vi "Measure Intensity Dep.vi"(0 "User Name":string, 1 "Cell details cluster":T3={"Cell Position"=16, "Cell Label"="", "Pixel to measure"=0, "Area (cm^2)"=0.126, "Variable"="", "Variable value"="", "Scan settings in queue"=0, "Light or dark"="", "Measurement type"=""} {"Pixel to measure" items=["All", "1", "2", "3", "4", "5", "6", "7", "8"]}, 2 "Date array":string[](array[string]), 5 "Experiment Title":string, 9 "No. of Suns":dbl, 11 "error in (no error)":errorcluster, 12 "Scan settings":T1={"J-V scan"=TRUE, "J-t scan"=FALSE, "Min voltage (V)"=0.0, "Max voltage (V)"=1.4, "Step (V)"=0.01, "Measurement delay (ms)"=10.0, "1st scan FB-SC"=TRUE, "Inverted structure"=FALSE, "Stabilisation time (s)"=0.0, "Stabilisation mode"=0, "Stabilisation value (V or A) "=0.0, "Step time (s)"=1.0, "Integration time"=0, "Repeat light scans"=FALSE, "Stabilisation in the dark?"=FALSE, "J-t Min (V)"=0.0, "J-t Max (V)"=1.4, "J-t Step (V)"=0.01, "Max. power stabilisation"=FALSE, "J-t 1st scan FB-SC"=TRUE, "J-t Inverted structure"=FALSE, "Max power tracking"=FALSE, "Vmp (V)"=0.7, "Total stabilisation time (s)"=100.0, "J-t best pixel only"=0, "Max power best pixel only"=0, "Vmp from J-V scan"=FALSE, "Intensity dependence"=FALSE, "P dep best pixel only"=0, "External quantum efficiency"=FALSE, "EQE best pixel only"=0, "WL min (nm)"=300.0, "WL max (nm)"=900.0, "WL step (nm)"=5.0, "Wait (ms)"=100.0, "No. of repeat scans"=2.0, "Only repeat for best pixel"=0, "Chopper Freq.  (Hz)"=90.0, "Time Constant (s)"=2.0, "Stabilisation time step (s)"=1.0, "Illumination conditions"=2, "Scan rate min (V/s)"=0.1, "Scan rate max (V/s)"=1.0, "No. of scan rate steps"=1.0, "Scan rate voltage step priority"=FALSE, "Scan rate measurement delay priority"=FALSE, "J-t Illumination conditions"=0, "White bias  (no. of suns)"=200.0, "Max P stab. Specific voltage"=FALSE} {"J-t Illumination conditions" items=["Light only", "Dark only", "Light then dark", "Dark then light"]; "No. of scan rate steps" min=1.0 step=1.0; "Illumination conditions" items=["Light only", "Dark only", "Light then dark", "Dark then light", "Light then dark then light", "Dark then light then dark"]; "Time Constant (s)" items=["0.003", "0.01", "0.03", "0.1", "0.3", "1", "3", "10", "30", "100"]; "Only repeat for best pixel" items=["only for best pixel", "for best 2 pixels", "for best 3 pixels", "for best 4 pixels", "for best 5 pixels", "for best 6 pixels", "for best 7 pixels", "for all pixels"]; "No. of repeat scans" min=1.0 step=1.0; "EQE best pixel only" items=["only the best pixel", "the best 2 pixel", "the best 3 pixel", "the best 4 pixel", "the best 5 pixel", "the best 6 pixel", "the best 7 pixel", "all pixels"]; "P dep best pixel only" items=["only the best pixel", "the best 2 pixels", "the best 3 pixels", "the best 4 pixels", "the best 5 pixels", "the best 6 pixels", "the best 7 pixels", "all pixels"]; "Max power best pixel only" items=["only the best pixel", "the best 2 pixels", "the best 3 pixels", "the best 4 pixels", "the best 5 pixels", "the best 6 pixels", "the best 7 pixels", "all pixels"]; "J-t best pixel only" items=["only the best pixel", "the best 2 pixels", "the best 3 pixels", "the best 4 pixels", "the best 5 pixels", "the best 6 pixels", "the best 7 pixels", "all pixels"]; "Integration time" items=["Fast", "Normal", "High Accuracy"]; "Stabilisation mode" items=["V", "I"]; "Measurement delay (ms)" min=10.0}, 13 "Scan rate (V/s)":dbl, 14 "Skip pixel?":bool) -> (4 "JV Curve":cluster{"Y":dbl[], "Y":dbl[]}[](graph), 15 "Log Table":string[][](table))   [LabVIEW 2016]
uses:
  TypeDefs/NPLC for JV scan.ctl
  <instrlib>/keithley_24xx/Keithley 24XX/Public/Data/Read (Single Point).vi
  TypeDefs/Settings Boolean.ctl
  TypeDefs/Scan settings.ctl
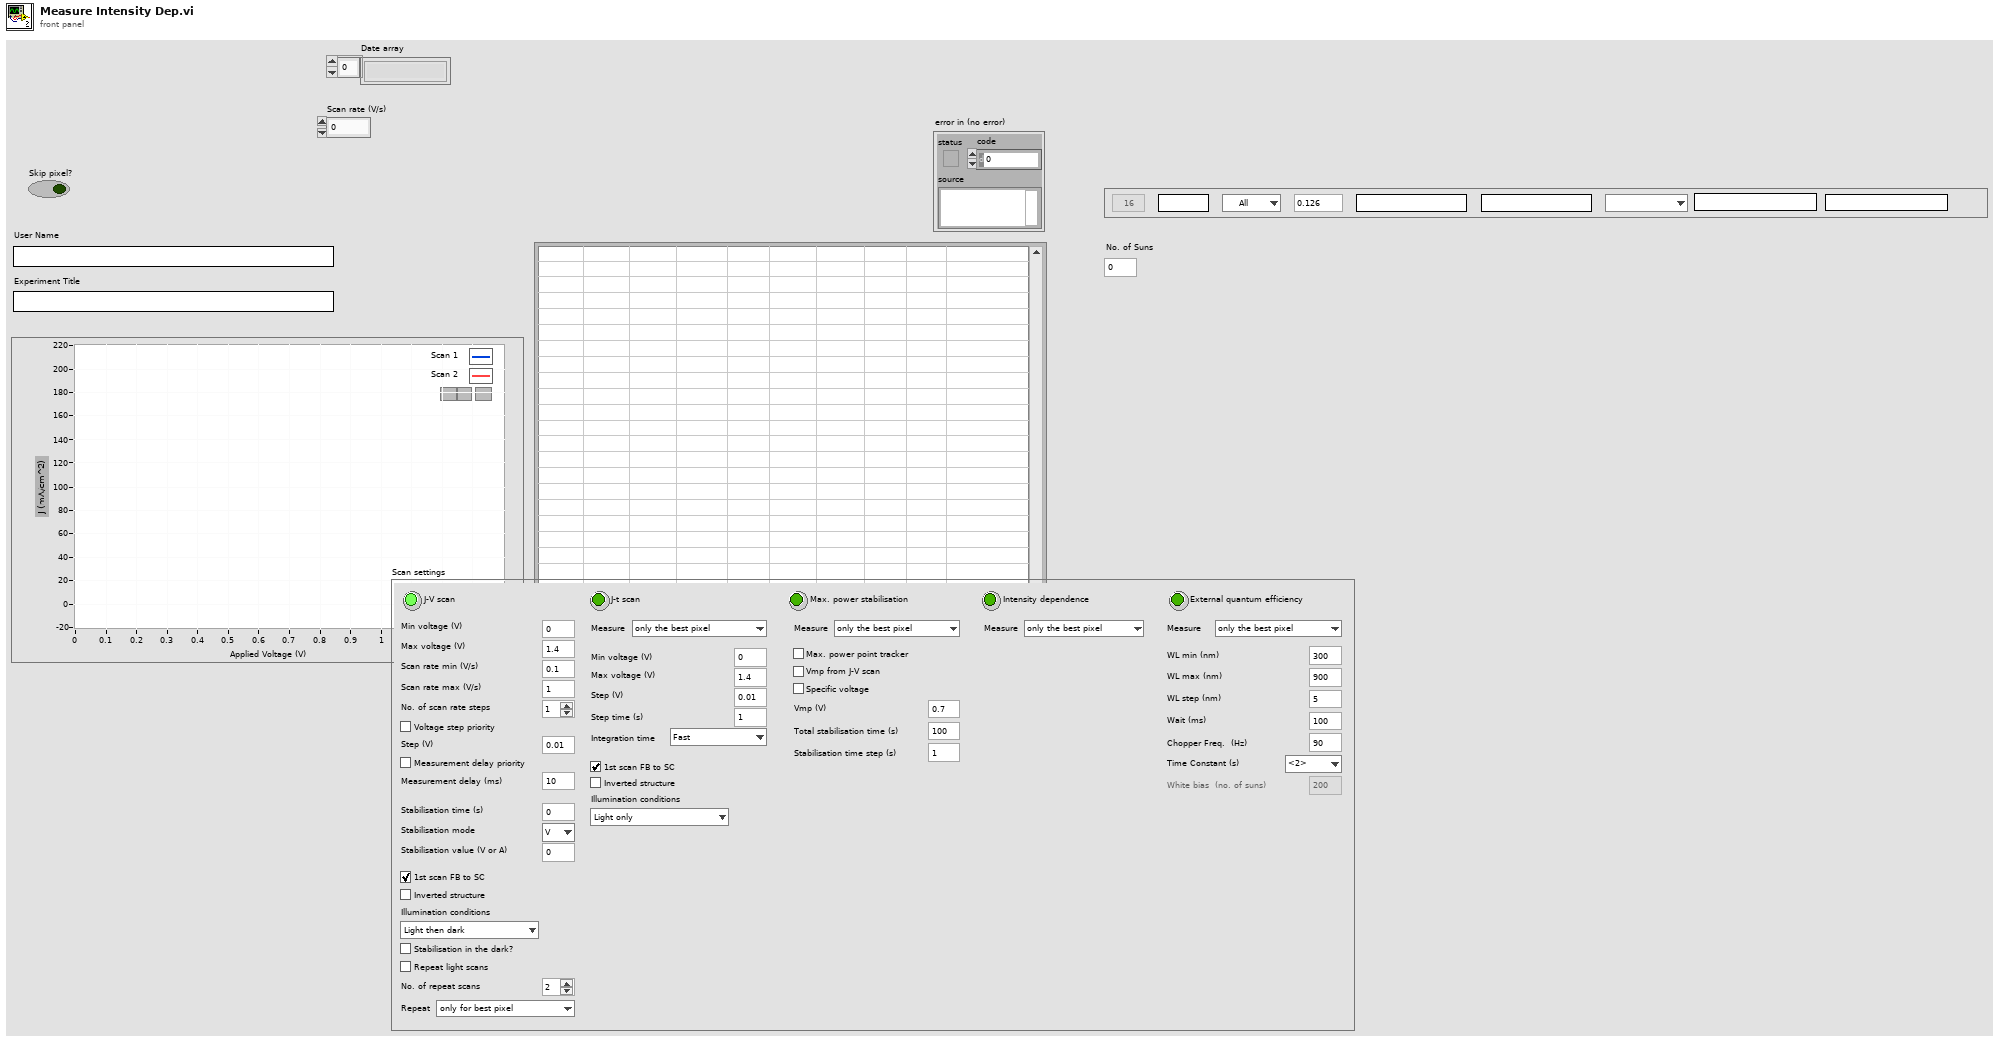
[diagram p1: front panel]
types:
  T1 = typedef "Scan settings.ctl" = cluster{"J-V scan":T2, "J-t scan":bool, "Min voltage (V)":dbl, "Max voltage (V)":dbl, "Step (V)":dbl, "Measurement delay (ms)":dbl, "1st scan FB-SC":bool, "Inverted structure":bool, "Stabilisation time (s)":dbl, "Stabilisation mode":u16, "Stabilisation value (V or A) ":dbl, "Step time (s)":dbl, "Integration time":u16, "Repeat light scans":bool, "Stabilisation in the dark?":bool, "J-t Min (V)":dbl, "J-t Max (V)":dbl, "J-t Step (V)":dbl, "Max. power stabilisation":bool, "J-t 1st scan FB-SC":bool, "J-t Inverted structure":bool, "Max power tracking":bool, "Vmp (V)":dbl, "Total stabilisation time (s)":dbl, "J-t best pixel only":u16, "Max power best pixel only":u16, "Vmp from J-V scan":bool, "Intensity dependence":bool, "P dep best pixel only":u16, "External quantum efficiency":bool, "EQE best pixel only":u16, "WL min (nm)":dbl, "WL max (nm)":dbl, "WL step (nm)":dbl, "Wait (ms)":dbl, "No. of repeat scans":dbl, "Only repeat for best pixel":u16, "Chopper Freq.  (Hz)":dbl, "Time Constant (s)":dbl, "Stabilisation time step (s)":dbl, "Illumination conditions":u16, "Scan rate min (V/s)":dbl, "Scan rate max (V/s)":dbl, "No. of scan rate steps":dbl, "Scan rate voltage step priority":bool, "Scan rate measurement delay priority":bool, "J-t Illumination conditions":u16, "White bias  (no. of suns)":dbl, "Max P stab. Specific voltage":bool}
  T2 = typedef "Settings Boolean.ctl" = bool
  T3 = cluster{"Cell Position":i32, "Cell Label":string, "Pixel to measure":u16, "Area (cm^2)":dbl, "Variable":string, "Variable value":string, "Scan settings in queue":u16, "Light or dark":string, "Measurement type":string}
  T4 = typedef "NPLC for JV scan.ctl" = dbl
  T5 = typedef "imagedata.ctl" = cluster{"image type":i32, "image depth":i32, "image":u8[], "mask":u8[], "colors":u32[], "Rectangle":cluster{"left":i16, "top":i16, "right":i16, "bottom":i16}}
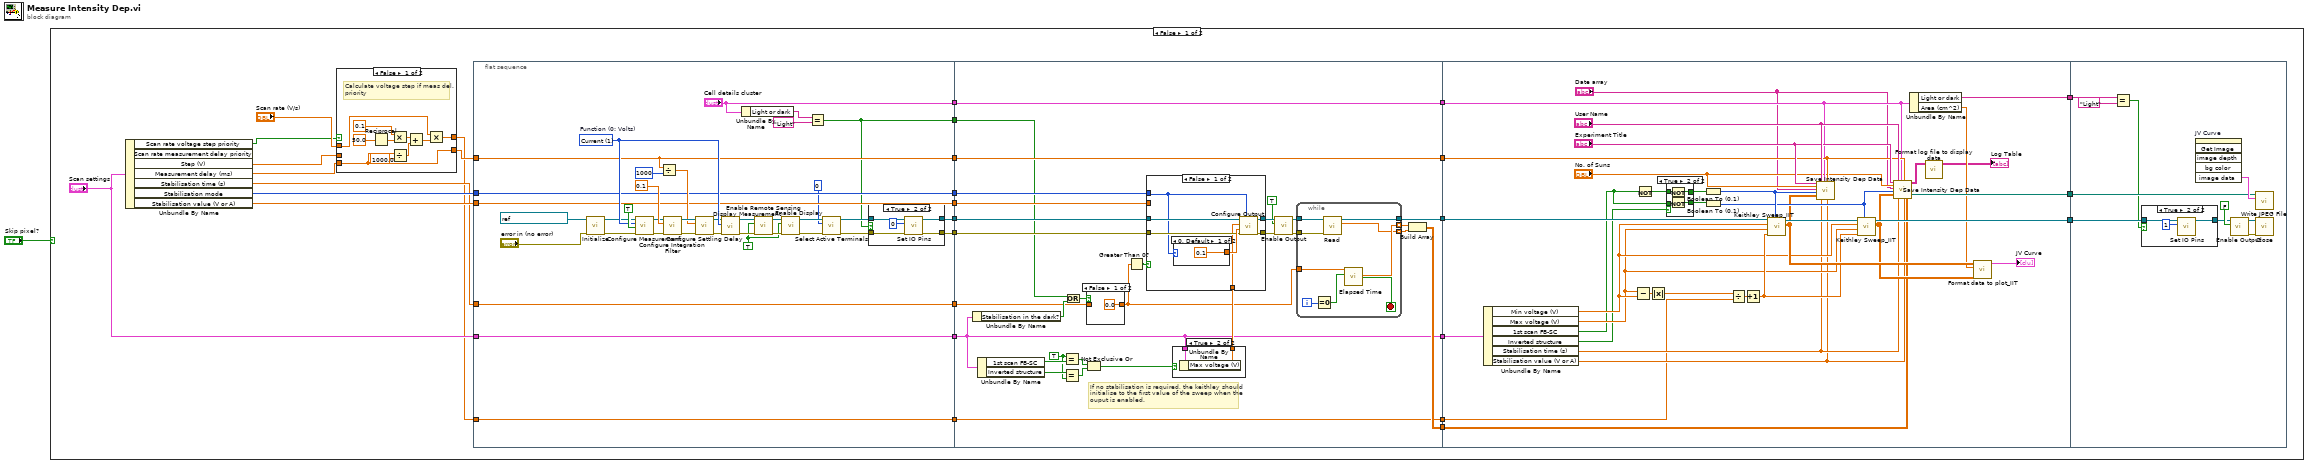
[diagram p0: block diagram]
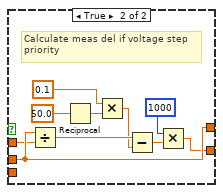
[diagram p2: hidden frame]
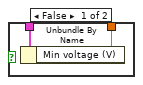
[diagram p5: hidden frame]
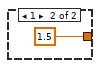
[diagram p6: hidden frame]
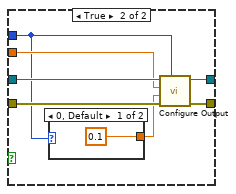
[diagram p7: hidden frame]
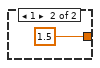
[diagram p8: hidden frame]
diagram:
  n1 = case shown="False" "Skip pixel?" {
    frame False {
      n2 = Unbundle By Name("Scan settings") -> ("Scan rate voltage step priority"=w2:bool, "Step (V)"=w6:dbl, "Measurement delay (ms)"=w5:dbl, "Stabilisation time (s)"=w8:dbl, "Stabilisation mode"=w10:u16, "Stabilisation value (V or A)"=w11:dbl)  [unwired: 1 out]
      n3 = case shown="False" w2 {
        tunnel: [w36 w44] -> w4
        tunnel: w5 -> [w36 _]
        tunnel: "Scan rate (V/s)" -> [w32 w41]
        tunnel: [w31 w50] -> w3
        tunnel: w6 -> [_ w50]
        frame False {
          # "Calculate voltage step if meas del.\npriority"
          n4 = Reciprocal(x=50.0) -> (1/x=w39:dbl)
          n5 = Multiply(x=T4 0.1, y=w39) -> (x*y=w37:T4)
          n6 = Divide(x=w36, y=1000.0) -> (x/y=w34:dbl)
          n7 = Add(x=w37, y=w34) -> (x+y=w33:T4)
          n8 = Multiply(x=w32, y=w33) -> (x*y=w31:T4)
        }
        frame True {
          # "Calculate meas del if voltage step\npriority"
          n9 = Divide(x=w50, y=w41) -> (x/y=w46:dbl)
          n10 = Reciprocal(x=50.0) -> (1/x=w48:dbl)
          n11 = Multiply(x=T4 0.1, y=w48) -> (x*y=w45:T4)
          n12 = Subtract(x=w46, y=w45) -> (x-y=w43:T4)
          n13 = Multiply(x=1000, y=w43) -> (x*y=w44:T4)
        }
      }
      n14 = flat-sequence {
        tunnel: [w68] -> w30
        tunnel: [w61] -> w29
        tunnel: [w62] -> w28
        tunnel: w11 -> [w68]
        tunnel: [w67] -> w27
        tunnel: w10 -> [w67]
        tunnel: [w66] -> w26
        tunnel: w8 -> [w66]
        tunnel: w4 -> [w65]
        tunnel: [w65] -> w25
        tunnel: [w64] -> w24
        tunnel: "Scan settings" -> [w64]
        tunnel: ["Cell details cluster"] -> w23
        tunnel: [w52] -> w22
        tunnel: w3 -> [w51]
        tunnel: [w51] -> w21
        tunnel: w30 -> [w113]
        tunnel: w29 -> [w121]
        tunnel: w28 -> [w122]
        tunnel: [w117] -> w20
        tunnel: [w114] -> w19
        tunnel: w27 -> [w110]
        tunnel: w26 -> [w99]
        tunnel: [w112] -> w18
        tunnel: w25 -> [w112]
        tunnel: [w97] -> w17
        tunnel: w24 -> [w97]
        tunnel: [w111] -> w16
        tunnel: w23 -> [w111]
        tunnel: w22 -> [w96]
        tunnel: [w95] -> w15
        tunnel: w21 -> [w95]
        tunnel: [w185] -> w14
        tunnel: [w178] -> w13
        tunnel: w20 -> [w192]
        tunnel: w19 -> [w177]
        tunnel: w18 -> [w174]
        tunnel: w17 -> [w173]
        tunnel: w16 -> [w167]
        tunnel: [w166] -> w12
        tunnel: w15 -> [w159]
        tunnel: w14 -> [w203]
        tunnel: w13 -> [w204]
        tunnel: w12 -> [w199]
        frame #0 {
          w69 = TRUE ("Enable Output (T: Enable)")
          w82 = u16 1 items=["Volts", "Current", "Resistance"]  # Function (0: Volts)
          n15 = call <instrlib>:"Initialize.vi"("error in (no error)"="error in (no error)", "VISA resource name"=refnum<visa-resource-name> "GPIB0::24::INSTR") -> ("error out"=w72:errorcluster, "VISA resource name out"=w73:refnum<visa-resource-name>)  [unwired: 3 in, 5 out]
          n16 = call <instrlib>:"Configure Measurement.vi"("error in (no error)"=w72, "Enable Auto Range (T:Enable)"=TRUE, "Function (0: Volts)"=w82, "VISA resource name"=w73) -> ("error out"=w75:errorcluster, "VISA resource name out"=w74:refnum<visa-resource-name>)  [unwired: 6 in]
          n17 = Divide(x=w65, y=1000) -> (x/y=w81:T4)
          n18 = call <instrlib>:"Configure Integration Filter.vi"("error in (no error)"=w75, "Measurement Speed (1 PLC)"=0.1, "VISA resource name"=w74) -> ("error out"=w84:errorcluster, "VISA resource name out"=w83:refnum<visa-resource-name>)  [unwired: 7 in]
          n19 = call <instrlib>:"Configure Settling Delay.vi"("error in (no error)"=w84, "Manual Settling Delay (0 sec)"=w81, "VISA resource name"=w83) -> ("error out"=w79:errorcluster, "VISA resource name out"=w78:refnum<visa-resource-name>)  [unwired: 7 in]
          n20 = call <instrlib>:"Display Measurement.vi"("error in (no error)"=w79, "Displayed Measurement (0: Voltage)"=w82, "VISA resource name"=w78) -> ("error out"=w77:errorcluster, "VISA resource name out"=w76:refnum<visa-resource-name>)  [unwired: 7 in]
          n21 = Unbundle By Name("Cell details cluster") -> ("Light or dark"=w60:string)
          n22 = call <instrlib>:"Enable Remote Sensing.vi"("error in (no error)"=w77, "Enable Remote Sensing (T: Enable)"=w69, "VISA resource name"=w76) -> ("error out"=w70:errorcluster, "VISA resource name out"=w71:refnum<visa-resource-name>)  [unwired: 7 in]
          n23 = call <instrlib>:"Enable Display.vi"("error in (no error)"=w70, "Enable Display (T: Enable)"=w69, "VISA resource name"=w71) -> ("error out"=w57:errorcluster, "VISA resource name out"=w58:refnum<visa-resource-name>)  [unwired: 7 in]
          n24 = Equal?(x=w60, y="Light") -> (x = y?=w52:bool)
          n25 = call <instrlib>:"Select Active Terminals.vi"("error in (no error)"=w57, "Active Terminals (0: Front)"=0, "VISA resource name"=w58) -> ("error out"=w55:errorcluster, "VISA resource name out"=w56:refnum<visa-resource-name>)  [unwired: 7 in]
          n26 = case shown="True" w52 {
            tunnel: w56 -> [w89 w93]
            tunnel: w55 -> [w88 w92]
            tunnel: [w89 w91] -> w62
            tunnel: [w88 w90] -> w61
            frame False {
            }
            frame True {
              n27 = call <instrlib>:"Set IO Pins.vi"("error in (no error)"=w92, "Output Pattern (0)"=0, "VISA resource name"=w93) -> ("error out"=w90:errorcluster, "VISA resource name out"=w91:refnum<visa-resource-name>)  [unwired: 7 in]
            }
          }
        }
        frame #1 {
          w106 = TRUE
          # "If no stabilisation is required, the keithley should\ninitialise to the first value of the sweep when the\nouput is enabled."
          n28 = Unbundle By Name(w97) -> ("Stabilisation in the dark?"=w101:bool)
          n29 = Unbundle By Name(w97) -> ("1st scan FB-SC"=w108:bool, "Inverted structure"=w107:bool)
          n30 = Equal?(x=w106, y=w108) -> (x = y?=w104:bool)
          n31 = Equal?(x=w107, y=w106) -> (x = y?=w103:bool)
          n32 = Or(x=w96, y=w101) -> (x .or. y?=w100:bool)
          n33 = Not Exclusive Or(1:w103, 2:w104) -> (0:w102:bool)
          n34 = case shown="False" w100 {
            tunnel: [0.0 ("Stabilisation time (s)") w126] -> w98
            tunnel: w99 -> [_ w126]
            frame False {
            }
            frame True {
            }
          }
          n35 = Greater Than 0?(x=w98) -> (x > 0?=w109:bool)
          n36 = case shown="True" w102 {
            tunnel: w97 -> [w127 w130]
            tunnel: [w128 w129] -> w105
            frame False {
              n37 = Unbundle By Name(w127) -> ("Min voltage (V)"=w128:dbl)
            }
            frame True {
              n38 = Unbundle By Name(w130) -> ("Max voltage (V)"=w129:dbl)
            }
          }
          n39 = case shown="False" w109 {
            tunnel: [w135 w146] -> w124
            tunnel: [w136 w145] -> w123
            tunnel: w122 -> [w133 w144]
            tunnel: w121 -> [w134 w143]
            tunnel: w113 -> [_ w142]
            tunnel: w110 -> [w132 w140]
            tunnel: w105 -> [w131 _]
            frame False {
              n40 = case shown="0, Default" w132 {
                tunnel: [0.1 1.5] -> w137
                frame 0, Default {
                }
                frame 1 {
                }
              }
              n41 = call <instrlib>:"Configure Output.vi"("Source Mode  (0: Voltage)"=w132, "error in (no error)"=w134, "Compliance  Level (0.1)"=w137, "Output Level (0)"=w131, "VISA resource name"=w133) -> ("error out"=w135:errorcluster, "VISA resource name out"=w136:refnum<visa-resource-name>)  [unwired: 5 in]
            }
            frame True {
              n42 = case shown="0, Default" w140 {
                tunnel: [0.1 1.5] -> w141
                frame 0, Default {
                }
                frame 1 {
                }
              }
              n43 = call <instrlib>:"Configure Output.vi"("Source Mode  (0: Voltage)"=w140, "error in (no error)"=w143, "Compliance  Level (0.1)"=w141, "Output Level (0)"=w142, "VISA resource name"=w144) -> ("error out"=w146:errorcluster, "VISA resource name out"=w145:refnum<visa-resource-name>)  [unwired: 5 in]
            }
          }
          n44 = call <instrlib>:"Enable Output.vi"("error in (no error)"=w124, "Enable Output (T: Enable)"=TRUE ("Output (Off)"), "VISA resource name"=w123) -> ("error out"=w118:errorcluster, "VISA resource name out"=w119:refnum<visa-resource-name>)  [unwired: 7 in]
          n45 = while {
            tunnel: w119 -> [w157]
            tunnel: w118 -> [w156]
            tunnel: [w155] -> w117
            tunnel: [w153] -> w116 mode=indexing
            tunnel: [w152] -> w115 mode=indexing
            tunnel: w98 -> [w149]
            i -> [w151]
            stop <- w154 stop-if-true
            n46 = Equal To 0?(x=w151) -> (x = 0?=w150:bool)
            n47 = call-poly <instrlib>:"Read.vi"("VISA resource name"=w157, "error in (no error)"=w156) -> ("VISA resource name out"=w155:refnum<visa-resource-name>, "Current"=w152:sgl)  [unwired: 7 in, 5 out]
            n48 = call "Elapsed Time"("Time Target (s)"=w149, "Reset"=w150) -> ("Elapsed Time (s)"=w153:dbl, "Time has Elapsed"=w154:bool)  [unwired: 10 in, 6 out]
          }
          n49 = Build Array(w116, w115) -> (w114:dbl[][])
        }
        frame #2 {
          n50 = Unbundle By Name(w173) -> ("Min voltage (V)"=w172:dbl, "Max voltage (V)"=w171:dbl, "1st scan FB-SC"=w161:bool, "Inverted structure"=w170:bool, "Stabilisation time (s)"=w169:dbl, "Stabilisation value (V or A)"=w168:dbl)
          n51 = Subtract(x=w171, y=w172) -> (x-y=w190:dbl)
          n52 = Not(x=w161) -> (.not. x?=w162:bool)
          n53 = Absolute Value(x=w190) -> (abs(x)=w191:dbl)
          n54 = case shown="True" w170 {
            tunnel: [w194 w198] -> w180
            tunnel: [w193 w197] -> w179
            tunnel: w161 -> [w193 w196]
            tunnel: w162 -> [w194 w195]
            frame False {
            }
            frame True {
              n55 = Not(x=w195) -> (.not. x?=w198:bool)
              n56 = Not(x=w196) -> (.not. x?=w197:bool)
            }
          }
          n57 = Boolean To (0,1)(Boolean=w180) -> (0, 1=w188:i16)
          n58 = Boolean To (0,1)(Boolean=w179) -> (0, 1=w186:i16)
          n59 = Divide(x=w191, y=w159) -> (x/y=w182:T4)
          n60 = Increment(x=w182) -> (x+1=w181:T4)
          n61 = call "Keithley Sweep_IIT.vi"("Sweep Direction"=w188, "Number of Points"=w181, "Maximum Amplitude"=w171, "Minimum Amplitude"=w172, "VISA resource name out 2"=w192) -> ("Data Array"=w184:dbl[][], "VISA resource name out"=w187:refnum<visa-resource-name>)  [unwired: 2 in, 1 out]
          n62 = call "Save Intensity Dep Data.vi"("Experiment Indicator"="Experiment Title", "No. of Suns"="No. of Suns", "Date array"="Date array", "Scan direction"=w188, "Data Array"=w184, "Username"="User Name", "Stabilisation time (ms)"=w169, "Cell details cluster"=w167, "Measurement Delay (ms)"=w174, "Stabilisation level \n(A or V depending on mode)"=w168) -> ()  [unwired: 6 in, 4 out]
          n63 = call "Keithley Sweep_IIT.vi"("Sweep Direction"=w186, "Number of Points"=w181, "Maximum Amplitude"=w171, "Minimum Amplitude"=w172, "VISA resource name out 2"=w187) -> ("Data Array"=w183:dbl[][], "VISA resource name out"=w185:refnum<visa-resource-name>)  [unwired: 2 in, 1 out]
          n64 = call "Save Intensity Dep Data.vi"("Experiment Indicator"="Experiment Title", "No. of Suns"="No. of Suns", "Date array"="Date array", "Scan direction"=w186, "Data Array"=w183, "Username"="User Name", "Stabilisation time (ms)"=w169, "Cell details cluster"=w167, "Measurement Delay (ms)"=w174, "Stabilisation level \n(A or V depending on mode)"=w168, "Stabilisation Data"=w177) -> ("Master Log"=w164:string[][], "File path for JV image"=w178:path)  [unwired: 5 in, 2 out]
          n65 = Unbundle By Name(w167) -> ("Light or dark"=w166:string, "Area (cm^2)"=w165:dbl)
          n66 = call "Format log file to display data.vi"("Master Log"=w164) -> ("Formatted table"=→"Log Table":string[][])  [unwired: 10 in]
          n67 = call "Format data to plot_IIT.vi"("Data Array 2"=w183, "Device Area (cm^2)"=w165, "Data Array"=w184) -> ("JV Curve"=→"JV Curve":cluster{"Y":dbl[], "Y":dbl[]}[])  [unwired: 8 in]
        }
        frame #3 {
          n68 = Equal?(x=w199, y="Light") -> (x = y?=w200:bool)
          n69 = case shown="True" w200 {
            tunnel: w203 -> [w209 w211]
            tunnel: [w209 w210] -> w202
            frame False {
            }
            frame True {
              n70 = call <instrlib>:"Set IO Pins.vi"("Output Pattern (0)"=1, "VISA resource name"=w211) -> ("VISA resource name out"=w210:refnum<visa-resource-name>)  [unwired: 8 in, 1 out]
            }
          }
          n71 = invoke on="JV Curve" class="XYGraph (strict)" method="Get Image"() -> ("image data"=w205:T5)  [unwired: 6 in, 5 out]
          n72 = call <instrlib>:"Enable Output.vi"("Enable Output (T: Enable)"=FALSE ("Output (Off)"), "VISA resource name"=w202) -> ("error out"=w207:errorcluster, "VISA resource name out"=w208:refnum<visa-resource-name>)  [unwired: 8 in]
          n73 = call <vilib>:"Write JPEG File.vi"("image data"=w205, "path to JPEG file"=w204) -> ()  [unwired: 8 in, 2 out]
          n74 = call <instrlib>:"Close.vi"("error in (no error)"=w207, "VISA resource name"=w208) -> ()  [unwired: 9 in, 1 out]
        }
      }
    }
    frame True {
    }
  }
